vi "Get Group Scalar GUID.vi"(7 "error in (no error)":errorcluster, 9 "name":string, 10 "item ref in":u64) -> (0 "error out":errorcluster, 2 "group scalar guid":string, 3 "item ref out":u64)   [LabVIEW 2018, in "FPGA Addon System Explorer.lvlib"]
uses:
  FPGA Addon System Explorer.lvlib
  NationalInstruments.VeriStand.SystemDefinitionAPI
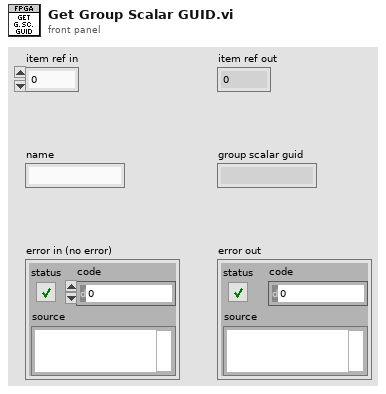
[diagram p1: front panel]
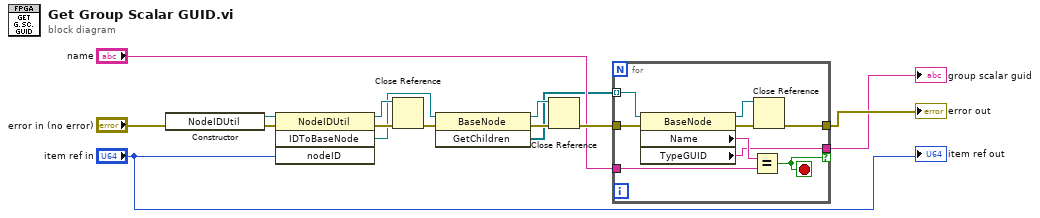
[diagram p0: block diagram]
diagram:
  n1 = constructor class="NodeIDUtil"(error in="error in (no error)") -> (reference out=w3:refnum<k24>, error out=w2:errorcluster)  [unwired: 2 in, 1 out]
  n2 = invoke class="NodeIDUtil" method="IDToBaseNode"(reference=w3, error in=w2, "nodeID"="item ref in") -> (reference out=w8:refnum<k24>, error out=w9:errorcluster, "IDToBaseNode"=w4:refnum<k24>)  [unwired: 1 in, 1 out]
  n3 = Close Reference(reference=w8, error in (no error)=w9) -> (error out=w10:errorcluster)
  n4 = invoke class="BaseNode" method="GetChildren"(reference=w4, error in=w10) -> (reference out=w12:refnum<k24>, error out=w11:errorcluster, "GetChildren"=w5:refnum<k24>[])  [unwired: 1 in]
  n5 = Close Reference(reference=w12, error in (no error)=w11) -> (error out=w13:errorcluster)
  n6 = for {
    tunnel: w13 -> [w24]
    tunnel: w5 -> [w23] mode=indexing
    tunnel: "name" -> [w21]
    tunnel: [w20] -> w7 if=w19
    tunnel: [w16] -> w14
    stop <- w19 stop-if-true
    n7 = property class="BaseNode"(reference=w23, error in=w24) -> (reference out=w17:refnum<k24>, error out=w18:errorcluster, "Name"=w22:string, "TypeGUID"=w20:string)
    n8 = Equal?(x=w22, y=w21) -> (x = y?=w19:bool)
    n9 = Close Reference(reference=w17, error in (no error)=w18) -> (error out=w16:errorcluster)
  }
  "error out" <- w14
  "group scalar guid" <- w7
  "item ref out" <- "item ref in"
